vi "Controle_des_lampe.vi"(0 "VISA resource name":refnum<visa-resource-name>, 1 "Status In":bool[](array[boolean])) -> (2 "VISA resource name dup":refnum<visa-resource-name>, 3 "Status Out":bool[](array[boolean]), 4 "String written":string)   [LabVIEW 2011]
panel:
  out "error out":errorcluster
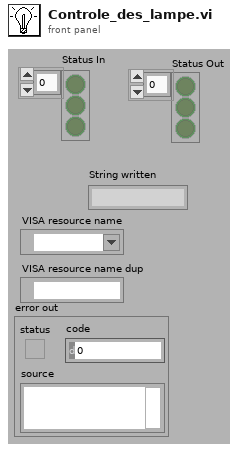
[diagram p1: front panel]
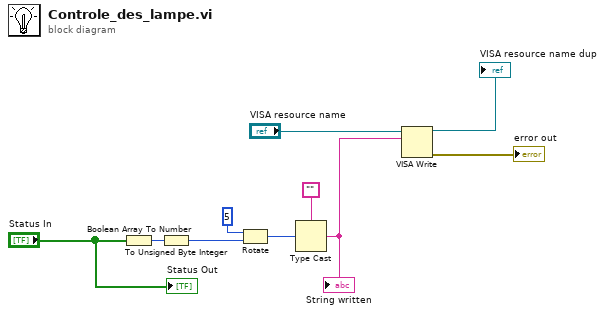
[diagram p0: block diagram]
diagram:
  n1 = Boolean Array To Number(Boolean array="Status In") -> (number=w9:u32)
  n2 = To Unsigned Byte Integer(number=w9) -> (unsigned 8bit integer=w7:u8)
  n3 = Rotate(1:w7, 2:u8 5 ("x")) -> (0:w6:u8)
  n4 = Type Cast(type="", x=w6) -> (*(type *) &x=w4:string)
  "String written" <- w4
  n5 = VISA Write(VISA resource name="VISA resource name", write buffer=w4) -> (VISA resource name out=→"VISA resource name dup":refnum<visa-resource-name>, error out=→"error out":errorcluster)  [unwired: 1 in, 1 out]
  "Status Out" <- "Status In"
